vi "练习 1.2.vi"() -> ()   [LabVIEW 2021]
panel:
  out "f2":dbl
  out "f1":dbl
  out "Waveform Graph":dynamicdata(graph)
  in  "stop":bool
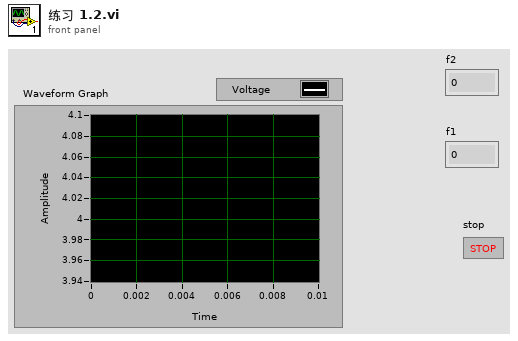
[diagram p1: front panel]
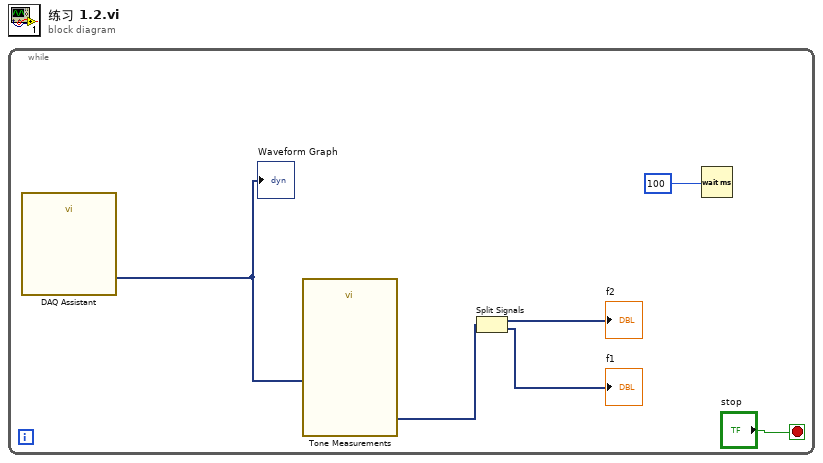
[diagram p0: block diagram]
diagram:
  n1 = while {
    stop <- "stop" stop-if-true
    n2 = call "DAQ Assistant"() -> ("data"=w2:dynamicdata)  [unwired: 17 in, 2 out]
    "Waveform Graph" <- w2
    n3 = call "Tone Measurements"("Signals"=w2) -> ("Frequency"=w4:dynamicdata)  [unwired: 9 in, 1 out]
    n4 = Split Signals(w4) -> (→"f2":dynamicdata, →"f1":dynamicdata)  [unwired: 2 in]
    n5 = Wait (ms)(milliseconds to wait=100) -> ()  [unwired: 1 out]
  }
